vi "close.vi"(8 "error in (no error)":errorcluster, 11 "CQT_DDS in":refnum<class "CQT_DDS.lvclass">) -> (0 "error out":errorcluster)   [LabVIEW 2011, in "CQT_DDS.lvclass"]
uses:
  CQT_DDS.lvclass
  CQT_DDS.lvclass/CQT_DDS.ctl
  C:/Program Files/National Instruments/LabVIEW 2011/instr.lib/CQT_DDS/DDSLibrary/20111109/CQTAD9958.dll
  Program Files/National Instruments/LabVIEW 2011/instr.lib/CQT_DDS/DDSLibrary/20111109/CQTAD9958.dll
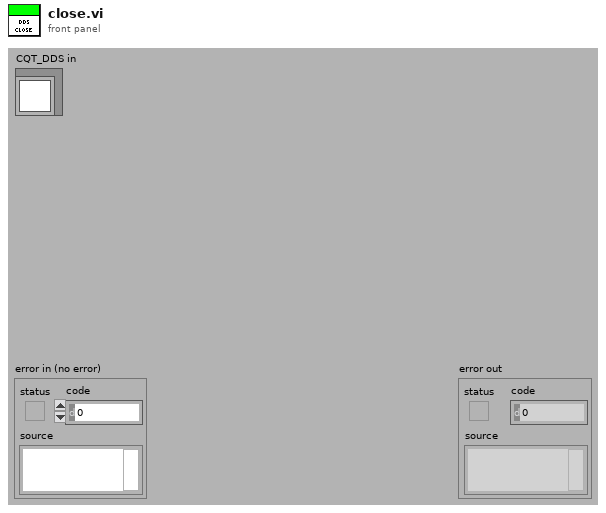
[diagram p1: front panel]
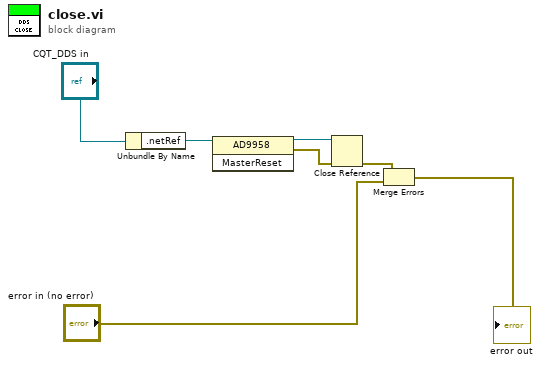
[diagram p0: block diagram]
diagram:
  n1 = Unbundle By Name("CQT_DDS in") -> (".netRef"=w6:refnum<k24>)
  n2 = invoke class="AD9958" method="MasterReset"(reference=w6) -> (reference out=w5:refnum<k24>, error out=w4:errorcluster)  [unwired: 2 in, 1 out]
  n3 = Close Reference(reference=w5, error in (no error)=w4) -> (error out=w3:errorcluster)
  n4 = Merge Errors(w3, "error in (no error)") -> (→"error out":errorcluster)
